vi "4.vi"   [LabVIEW 2015]
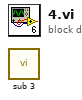
[diagram p0: block diagram]
diagram:
  n1 = call "sub 3.vi"() -> ()  [unwired: 10 in, 2 out]
